vi "Servo_find_index.vi"(9 "PWM":T1 items=["Invalid"=0, "PWM1"=1, "PWM2"=2, "PWM9"=9, "PWM10"=10]) -> (0 "Array":cluster{"value":dbl}[](array[cluster]), 1 "value 3":dbl, 2 "value 2":dbl, 3 "value":dbl)   [LabVIEW 2009, in "Servo.lvlib"]
uses:
  Servo.lvlib
  PWM/PWM_Name.ctl
  Servo_global_test.vi
  PWM.lvlib
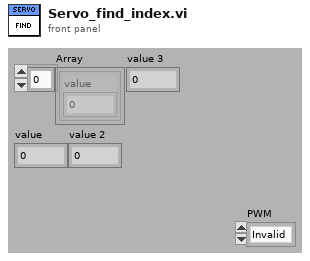
[diagram p1: front panel]
types:
  T1 = typedef "PWM.lvlib/PWM_Name.ctl" = u16
  T2 = cluster{"String":string, cluster{"value":dbl}[]}[]
  T3 = cluster{"[0]":cluster{"value":dbl}, "[1]":cluster{"value":dbl}, "[2]":cluster{"value":dbl}}
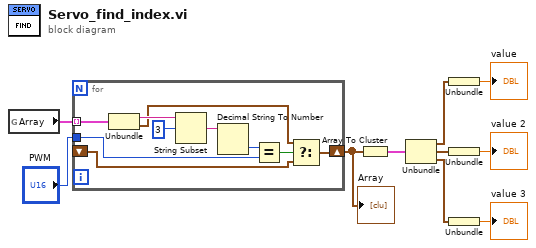
[diagram p0: block diagram]
diagram:
  n1 = global read "Servo_global_test.vi" "Array"() -> (w9:T2)
  n2 = for {
    tunnel: w9 -> [w20] mode=indexing
    tunnel: "PWM" -> [w16]
    shift-right: [w13] -> w8
    shift-left: _ -> [w12]
    n3 = Unbundle(w20) -> ("String"=w19:string, w15:cluster{"value":dbl}[])
    n4 = String Subset(string=w19, offset (0)=3) -> (substring=w17:string)  [unwired: 1 in]
    n5 = Decimal String To Number(string=w17) -> (number=w11:i32)  [unwired: 2 in, 1 out]
    n6 = Equal?(x=w11, y=w16) -> (x = y?=w14:bool)
    n7 = Select(t=w15, s=w14, f=w12) -> (s? t:f=w13:cluster{"value":dbl}[])
  }
  "Array" <- w8
  n8 = Array To Cluster(array=w8) -> (cluster=w7:T3)
  n9 = Unbundle(w7) -> ("[0]"=w6:cluster{"value":dbl}, "[1]"=w5:cluster{"value":dbl}, "[2]"=w4:cluster{"value":dbl})
  n10 = Unbundle(w6) -> ("value"=→"value":dbl)
  n11 = Unbundle(w5) -> ("value"=→"value 2":dbl)
  n12 = Unbundle(w4) -> ("value"=→"value 3":dbl)
